vi "dfd_FLP Lattice Basic Section.vi"(2 "k(m)":dbl format="%.2f", 3 "w(m-1)":dbl format="%.2f", 4 "x(m)":dbl format="%.2f") -> (0 "w(m)":dbl format="%.2f", 1 "x(m-1)":dbl format="%.2f")   [LabVIEW 2017, in "NI_DigFilter_FXP.lvlib"]
uses:
  <vilib>/addons/Digital Filter Design/NI_DigFilter_FXP.lvlib
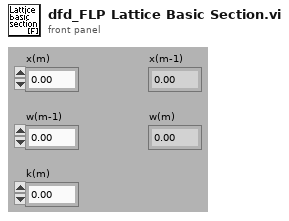
[diagram p1: front panel]
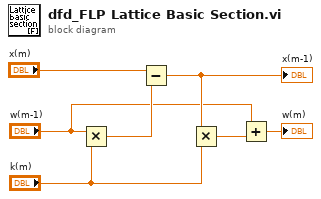
[diagram p0: block diagram]
diagram:
  n1 = Multiply(x="w(m-1)", y="k(m)") -> (x*y=w6:dbl)
  n2 = Subtract(x="x(m)", y=w6) -> (x-y=w4:dbl)
  "x(m-1)" <- w4
  n3 = Multiply(x=w4, y="k(m)") -> (x*y=w3:dbl)
  n4 = Add(x="w(m-1)", y=w3) -> (x+y=→"w(m)":dbl)
